vi "SCPI_read_numeric.vi"(0 "VISA":refnum<visa-resource-name>, 1 "SCIPI":T1 items=["*IDN?", "*SAV 1", "*RCL 1", "INSTTrument CH1", "INSTTrument CH2", "INSTrument?", "MEASure:CURRent? CH1", "MEASure:CURRent? CH2", "MEASure:VOLTage? CH1", "MEASure:VOLTage? CH2", "MEASure:POWEr? CH1", "MEASure:POWEr? CH2", "CH1:CURRent?", "CH2:CURRent?", "CH1:VOLTage? ", "CH2:VOLTage? ", "OUTPut CH1,ON", "OUTPut CH1,OFF", "OUTPut CH2,ON", "OUTPut CH2,OFF", "OUTPut CH3,ON", "OUTPut CH3,OFF", "OUTPut:TRACK 0", "OUTPut:TRACK 1", "OUTPut:TRACK 2", "OUTPut:WAVE CH1,ON", "OUTPut:WAVE CH1,OFF", "OUTPut:WAVE CH2,ON", "OUTPut:WAVE CH2,OFF"], 2 "error in (no error)":errorcluster) -> (3 "VISA resource name out":refnum<visa-resource-name>, 4 "read buffer - string":string, 5 "numeric value":dbl, 6 "error out":errorcluster)   [LabVIEW 2020]
doc: "Wysyłanie podstawowych komend SCPI - zasilacz SIGLENT SPD3303X-E"
uses:
  controls/SCPI_enum.ctl
panel:
  in  "byte count":u32=4096
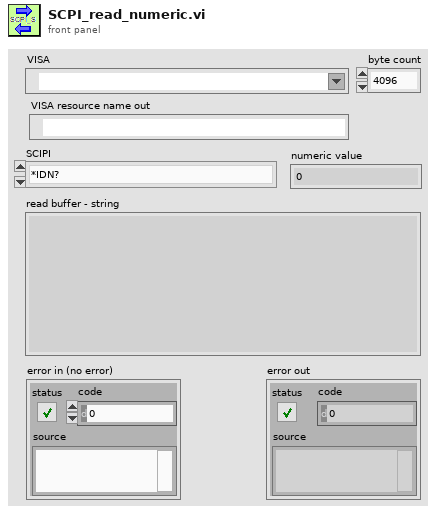
[diagram p1: front panel]
types:
  T1 = typedef "SCPI_enum.ctl" = u16
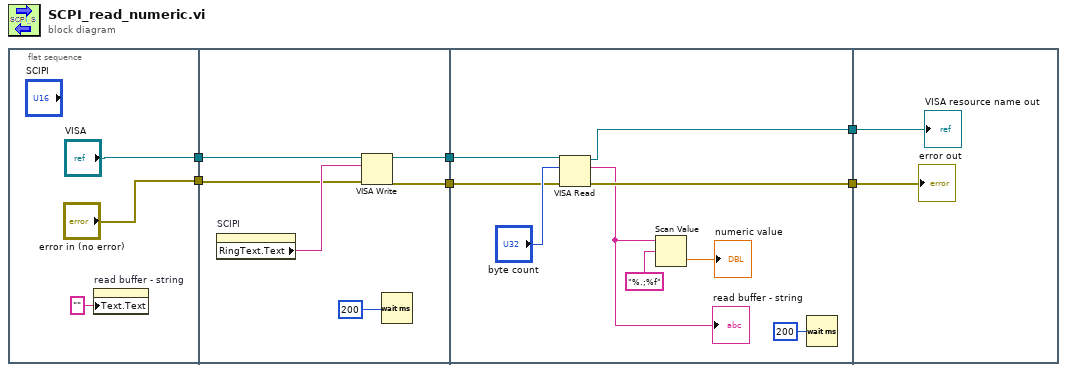
[diagram p0: block diagram]
diagram:
  n1 = flat-sequence {
    tunnel: ["VISA"] -> w6
    tunnel: ["error in (no error)"] -> w2
    tunnel: w6 -> [w13]
    tunnel: [w12] -> w4
    tunnel: [w11] -> w3
    tunnel: w2 -> [w10]
    tunnel: [w22] -> w5
    tunnel: w4 -> [w21]
    tunnel: w3 -> [w20]
    tunnel: [w19] -> w1
    tunnel: w5 -> [w26]
    tunnel: w1 -> [w25]
    frame #0 {
      n2 = property on="read buffer - string" class="Str"("Text.Text"="") -> ()  [unwired: 2 in, 2 out]
    }
    frame #1 {
      n3 = property on="SCIPI" class="Ring (strict)"() -> ("RingText.Text"=w15:string)  [unwired: 2 in, 2 out]
      n4 = VISA Write(VISA resource name=w13, write buffer=w15, error in (no error)=w10) -> (VISA resource name out=w12:refnum<visa-resource-name>, error out=w11:errorcluster)  [unwired: 1 out]
      n5 = Wait (ms)(milliseconds to wait=u32 200) -> ()  [unwired: 1 out]
    }
    frame #2 {
      n6 = VISA Read(VISA resource name=w21, byte count="byte count", error in (no error)=w20) -> (VISA resource name out=w19:refnum<visa-resource-name>, read buffer=w16:string, error out=w22:errorcluster)  [unwired: 1 out]
      "read buffer - string" <- w16
      n7 = Scan Value(string=w16, format string="%.;%f") -> (value=→"numeric value":dbl)  [unwired: 1 in, 1 out]
      n8 = Wait (ms)(milliseconds to wait=u32 200) -> ()  [unwired: 1 out]
    }
    frame #3 {
      "error out" <- w26
      "VISA resource name out" <- w25
    }
  }
